vi "RtdeInitialize.vi"(0 "error in":errorcluster, 5 "Frequency":dbl, 6 "InputData":i32[](array[ring]) items=["SpeedSliderMask", "SpeedSliderFraction", "StandardDigitalOutputMask", "ConfigurableDigitalOutputMask", "StandardDigitalOutput", "ConfigurableDigitalOutput", "StandardAnalogOutputMask", "StandardAnalogOutputType", "StandardAnalogOutput0", "StandardAnalogOutput1", "InputBtRegisters0To31", "InputBtRegisters32To63", "InputBitRegisters", "InputIntRegisters", "InputDoubleRegisters", "ExternalForceTorque"], 7 "OutputData":i32[](array[ring]) items=["Timestamp", "TargetQ", "TargetQd", "TargetQdd", "TargetCurrent", "TargetMoment", "ActualQ", "ActualQd", "ActualCurrent", "JointControlOutput", "ActualTcpPose", "ActualTcpSpeed", "ActualTcpForce", "TargetTcpPose", "TargetTcpSpeed", "ActualDigitalInputBits", "JointTemperatures", "ActualExecutionTime", "RobotMode", "JointMode", "SafetyMode", "SafetyStatus", "ActualToolAccelerometer", "SpeedScaling", "TargetSpeedFraction", "ActualMomentum", "ActualMainVoltage", "ActualRobotVoltage", "ActualRobotCurrent", "ActualJointVoltage", "ActualDigitalOutputBits", "RuntimeState", "ElbowPosition", "ElbowVelocity", "RobotStatusBits", "SafetyStatusBits", "AnalogIOTypes", "StandardAnalogInput0", "StandardAnalogInput1", "StandardAnalogOutput0", "StandardAnalogOutput1", "IOCurrent", "Euromap67InputBits", "Euromap67OutputBits", "Euromap67_24VVoltage", "Euromap67_24VCurrent", "ToolMode", "ToolAnalogInputTypes", "ToolAnalogInput0", "ToolAnalogInput1", "ToolOutputVoltage", "ToolOutputCurrent", "ToolTemperature", "TcpForceScalar", "OutputBitRegisters0To31", "OutputBitRegisters32To63", "OutputBitRegisters", "OutputIntRegisters", "OutputDoubleRegisters", "InputBitRegisters0To31", "InputBitRegisters32To63", "InputBitRegisters", "InputIntRegisters", "InputDoubleRegisters", "ToolOutputMode", "ToolDigitalOutput0mode", "ToolDigitalOutput1Mode", "Payload", "PayloadCOG", "PayloadInertia", "ScriptControlLine", "FTRawWrench"], 8 "InputBitRegisters":i32[](array[numeric]), 9 "OutputBitRegisters":i32[](array[numeric]), 10 "InputIntRegisters":i32[](array[numeric]), 11 "OutputIntRegisters":i32[](array[numeric]), 12 "InputDoubleRegisters":i32[](array[numeric]), 13 "OutputDoubleRegisters":i32[](array[numeric])) -> (14 "error out":errorcluster, 19 "RTDE Connect Parameters":refnum<k24>)   [LabVIEW 2016, in "UnderAutomation.UniversalRobots.lvlib"]
uses:
  UnderAutomation.UniversalRobots.lvlib
  C:/Users/fg/Documents/UniversalRobots.vi/LabVIEW_2024/UnderAutomation.UniversalRobots/lib/UnderAutomation.UniversalRobots.dll
  LabVIEW_2024/UnderAutomation.UniversalRobots/lib/UnderAutomation.UniversalRobots.dll
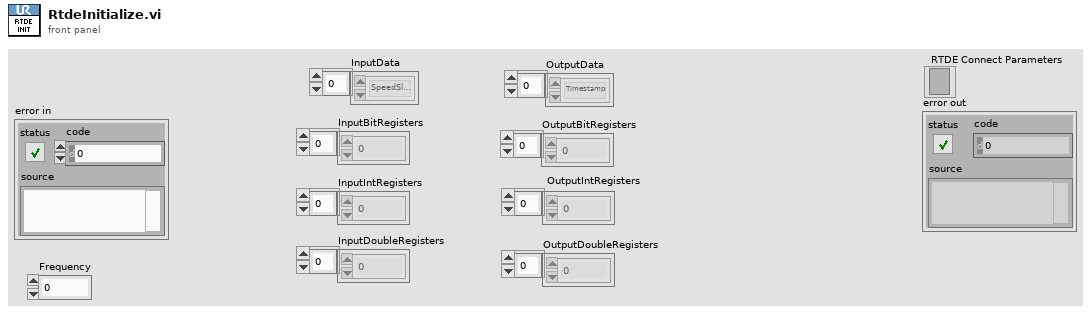
[diagram p1: front panel]
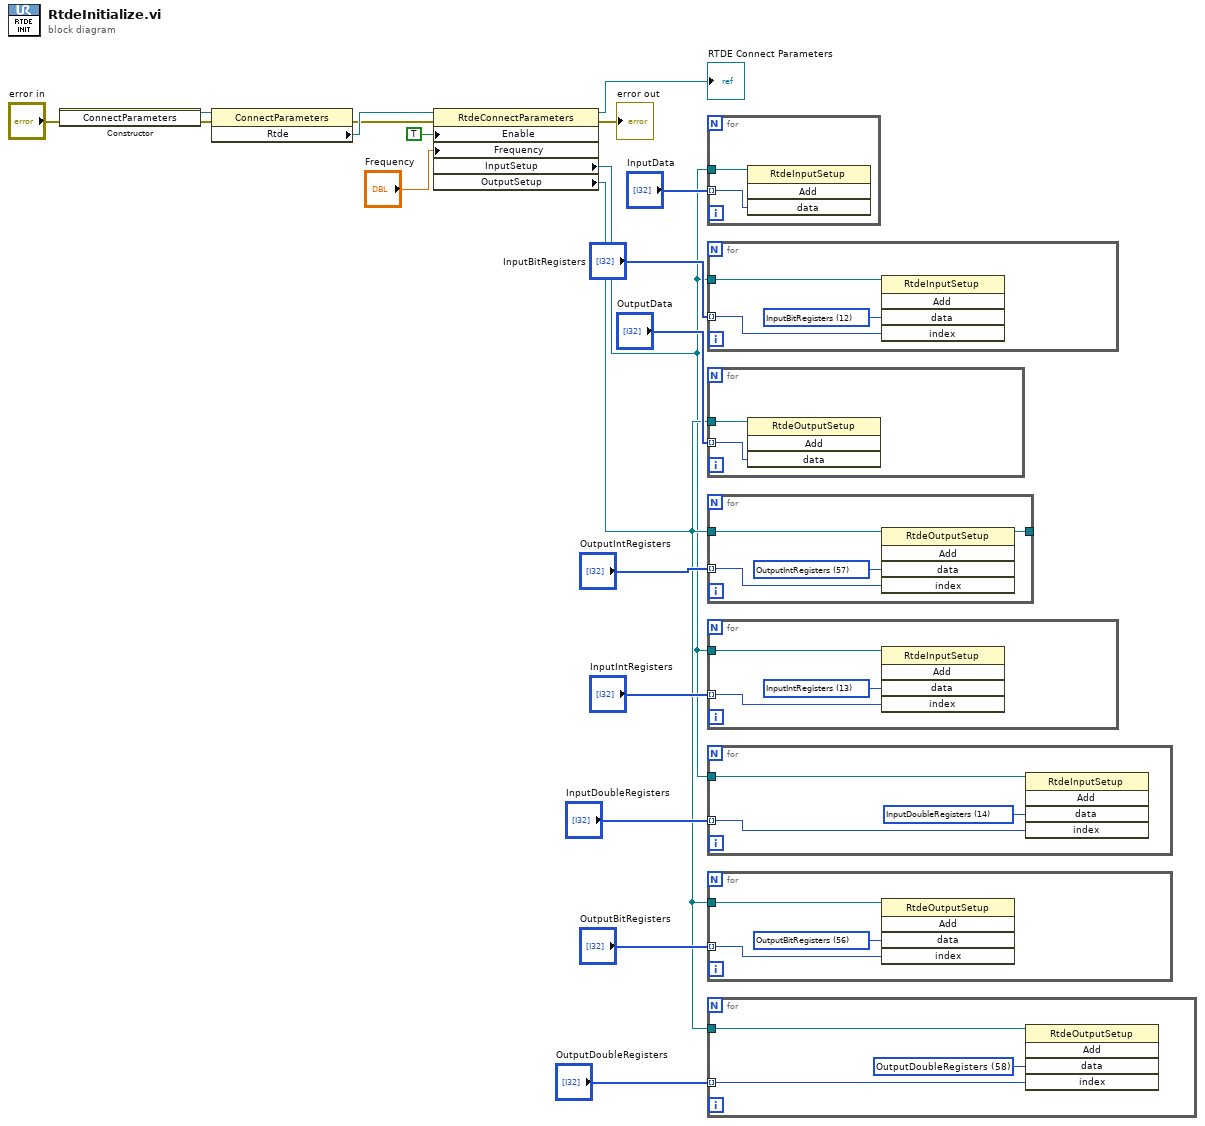
[diagram p0: block diagram]
diagram:
  n1 = constructor class="ConnectParameters"(error in="error in") -> (reference out=w19:refnum<k24>, error out=w15:errorcluster)  [unwired: 2 in, 1 out]
  n2 = property class="ConnectParameters"(reference=w19, error in=w15) -> (error out=w14:errorcluster, "Rtde"=w18:refnum<k24>)  [unwired: 1 out]
  n3 = property class="RtdeConnectParameters"(reference=w18, error in=w14, "Enable"=TRUE, "Frequency"="Frequency") -> (reference out=→"RTDE Connect Parameters":refnum<k24>, error out=→"error out":errorcluster, "InputSetup"=w1:refnum<k24>, "OutputSetup"=w2:refnum<k24>)
  n4 = for {
    tunnel: w1 -> [w21]
    tunnel: "InputData" -> [w20] mode=indexing
    n5 = invoke class="RtdeInputSetup" method="Add"(reference=w21, "data"=w20) -> ()  [unwired: 2 in, 4 out]
  }
  n6 = for {
    tunnel: w1 -> [w24]
    tunnel: "InputBitRegisters" -> [w22] mode=indexing
    w23 = 12 items=["SpeedSliderMask", "SpeedSliderFraction", "StandardDigitalOutputMask", "ConfigurableDigitalOutputMask", "StandardDigitalOutput", "ConfigurableDigitalOutput", "StandardAnalogOutputMask", "StandardAnalogOutputType", "StandardAnalogOutput0", "StandardAnalogOutput1", "InputBtRegisters0To31", "InputBtRegisters32To63", "InputBitRegisters", "InputIntRegisters", "InputDoubleRegisters", "ExternalForceTorque"] ("data")
    n7 = invoke class="RtdeInputSetup" method="Add"(reference=w24, "data"=w23, "index"=w22) -> ()  [unwired: 2 in, 5 out]
  }
  n8 = for {
    tunnel: w2 -> [w26]
    tunnel: "OutputData" -> [w25] mode=indexing
    n9 = invoke class="RtdeOutputSetup" method="Add"(reference=w26, "data"=w25) -> ()  [unwired: 2 in, 4 out]
  }
  n10 = for {
    tunnel: w2 -> [w30]
    tunnel: "OutputIntRegisters" -> [w28] mode=indexing
    tunnel: [w29] -> _
    w27 = 57 items=["Timestamp", "TargetQ", "TargetQd", "TargetQdd", "TargetCurrent", "TargetMoment", "ActualQ", "ActualQd", "ActualCurrent", "JointControlOutput", "ActualTcpPose", "ActualTcpSpeed", "ActualTcpForce", "TargetTcpPose", "TargetTcpSpeed", "ActualDigitalInputBits", "JointTemperatures", "ActualExecutionTime", "RobotMode", "JointMode", "SafetyMode", "SafetyStatus", "ActualToolAccelerometer", "SpeedScaling", "TargetSpeedFraction", "ActualMomentum", "ActualMainVoltage", "ActualRobotVoltage", "ActualRobotCurrent", "ActualJointVoltage", "ActualDigitalOutputBits", "RuntimeState", "ElbowPosition", "ElbowVelocity", "RobotStatusBits", "SafetyStatusBits", "AnalogIOTypes", "StandardAnalogInput0", "StandardAnalogInput1", "StandardAnalogOutput0", "StandardAnalogOutput1", "IOCurrent", "Euromap67InputBits", "Euromap67OutputBits", "Euromap67_24VVoltage", "Euromap67_24VCurrent", "ToolMode", "ToolAnalogInputTypes", "ToolAnalogInput0", "ToolAnalogInput1", "ToolOutputVoltage", "ToolOutputCurrent", "ToolTemperature", "TcpForceScalar", "OutputBitRegisters0To31", "OutputBitRegisters32To63", "OutputBitRegisters", "OutputIntRegisters", "OutputDoubleRegisters", "InputBitRegisters0To31", "InputBitRegisters32To63", "InputBitRegisters", "InputIntRegisters", "InputDoubleRegisters", "ToolOutputMode", "ToolDigitalOutput0mode", "ToolDigitalOutput1Mode", "Payload", "PayloadCOG", "PayloadInertia", "ScriptControlLine", "FTRawWrench"] ("data")
    n11 = invoke class="RtdeOutputSetup" method="Add"(reference=w30, "data"=w27, "index"=w28) -> (reference out=w29:refnum<k24>)  [unwired: 2 in, 4 out]
  }
  n12 = for {
    tunnel: w1 -> [w33]
    tunnel: "InputIntRegisters" -> [w31] mode=indexing
    w32 = 13 items=["SpeedSliderMask", "SpeedSliderFraction", "StandardDigitalOutputMask", "ConfigurableDigitalOutputMask", "StandardDigitalOutput", "ConfigurableDigitalOutput", "StandardAnalogOutputMask", "StandardAnalogOutputType", "StandardAnalogOutput0", "StandardAnalogOutput1", "InputBtRegisters0To31", "InputBtRegisters32To63", "InputBitRegisters", "InputIntRegisters", "InputDoubleRegisters", "ExternalForceTorque"] ("data")
    n13 = invoke class="RtdeInputSetup" method="Add"(reference=w33, "data"=w32, "index"=w31) -> ()  [unwired: 2 in, 5 out]
  }
  n14 = for {
    tunnel: w1 -> [w36]
    tunnel: "InputDoubleRegisters" -> [w34] mode=indexing
    w35 = 14 items=["SpeedSliderMask", "SpeedSliderFraction", "StandardDigitalOutputMask", "ConfigurableDigitalOutputMask", "StandardDigitalOutput", "ConfigurableDigitalOutput", "StandardAnalogOutputMask", "StandardAnalogOutputType", "StandardAnalogOutput0", "StandardAnalogOutput1", "InputBtRegisters0To31", "InputBtRegisters32To63", "InputBitRegisters", "InputIntRegisters", "InputDoubleRegisters", "ExternalForceTorque"] ("data")
    n15 = invoke class="RtdeInputSetup" method="Add"(reference=w36, "data"=w35, "index"=w34) -> ()  [unwired: 2 in, 5 out]
  }
  n16 = for {
    tunnel: w2 -> [w39]
    tunnel: "OutputBitRegisters" -> [w38] mode=indexing
    w37 = 56 items=["Timestamp", "TargetQ", "TargetQd", "TargetQdd", "TargetCurrent", "TargetMoment", "ActualQ", "ActualQd", "ActualCurrent", "JointControlOutput", "ActualTcpPose", "ActualTcpSpeed", "ActualTcpForce", "TargetTcpPose", "TargetTcpSpeed", "ActualDigitalInputBits", "JointTemperatures", "ActualExecutionTime", "RobotMode", "JointMode", "SafetyMode", "SafetyStatus", "ActualToolAccelerometer", "SpeedScaling", "TargetSpeedFraction", "ActualMomentum", "ActualMainVoltage", "ActualRobotVoltage", "ActualRobotCurrent", "ActualJointVoltage", "ActualDigitalOutputBits", "RuntimeState", "ElbowPosition", "ElbowVelocity", "RobotStatusBits", "SafetyStatusBits", "AnalogIOTypes", "StandardAnalogInput0", "StandardAnalogInput1", "StandardAnalogOutput0", "StandardAnalogOutput1", "IOCurrent", "Euromap67InputBits", "Euromap67OutputBits", "Euromap67_24VVoltage", "Euromap67_24VCurrent", "ToolMode", "ToolAnalogInputTypes", "ToolAnalogInput0", "ToolAnalogInput1", "ToolOutputVoltage", "ToolOutputCurrent", "ToolTemperature", "TcpForceScalar", "OutputBitRegisters0To31", "OutputBitRegisters32To63", "OutputBitRegisters", "OutputIntRegisters", "OutputDoubleRegisters", "InputBitRegisters0To31", "InputBitRegisters32To63", "InputBitRegisters", "InputIntRegisters", "InputDoubleRegisters", "ToolOutputMode", "ToolDigitalOutput0mode", "ToolDigitalOutput1Mode", "Payload", "PayloadCOG", "PayloadInertia", "ScriptControlLine", "FTRawWrench"] ("data")
    n17 = invoke class="RtdeOutputSetup" method="Add"(reference=w39, "data"=w37, "index"=w38) -> ()  [unwired: 2 in, 5 out]
  }
  n18 = for {
    tunnel: w2 -> [w42]
    tunnel: "OutputDoubleRegisters" -> [w41] mode=indexing
    w40 = 58 items=["Timestamp", "TargetQ", "TargetQd", "TargetQdd", "TargetCurrent", "TargetMoment", "ActualQ", "ActualQd", "ActualCurrent", "JointControlOutput", "ActualTcpPose", "ActualTcpSpeed", "ActualTcpForce", "TargetTcpPose", "TargetTcpSpeed", "ActualDigitalInputBits", "JointTemperatures", "ActualExecutionTime", "RobotMode", "JointMode", "SafetyMode", "SafetyStatus", "ActualToolAccelerometer", "SpeedScaling", "TargetSpeedFraction", "ActualMomentum", "ActualMainVoltage", "ActualRobotVoltage", "ActualRobotCurrent", "ActualJointVoltage", "ActualDigitalOutputBits", "RuntimeState", "ElbowPosition", "ElbowVelocity", "RobotStatusBits", "SafetyStatusBits", "AnalogIOTypes", "StandardAnalogInput0", "StandardAnalogInput1", "StandardAnalogOutput0", "StandardAnalogOutput1", "IOCurrent", "Euromap67InputBits", "Euromap67OutputBits", "Euromap67_24VVoltage", "Euromap67_24VCurrent", "ToolMode", "ToolAnalogInputTypes", "ToolAnalogInput0", "ToolAnalogInput1", "ToolOutputVoltage", "ToolOutputCurrent", "ToolTemperature", "TcpForceScalar", "OutputBitRegisters0To31", "OutputBitRegisters32To63", "OutputBitRegisters", "OutputIntRegisters", "OutputDoubleRegisters", "InputBitRegisters0To31", "InputBitRegisters32To63", "InputBitRegisters", "InputIntRegisters", "InputDoubleRegisters", "ToolOutputMode", "ToolDigitalOutput0mode", "ToolDigitalOutput1Mode", "Payload", "PayloadCOG", "PayloadInertia", "ScriptControlLine", "FTRawWrench"] ("data")
    n19 = invoke class="RtdeOutputSetup" method="Add"(reference=w42, "data"=w40, "index"=w41) -> ()  [unwired: 2 in, 5 out]
  }
